vi "Flatten.vi"(8 "error in":errorcluster, 9 "Data":T1) -> (0 "error out":errorcluster, 2 "Buffer":u8[](array[numeric]) format="%.0x")   [LabVIEW 2020, in "TcpPayload.lvlib"]
uses:
  TcpPayload.lvlib
  Data.ctl
  lv-protoc/LV-Proto/LV-Proto.lvlib
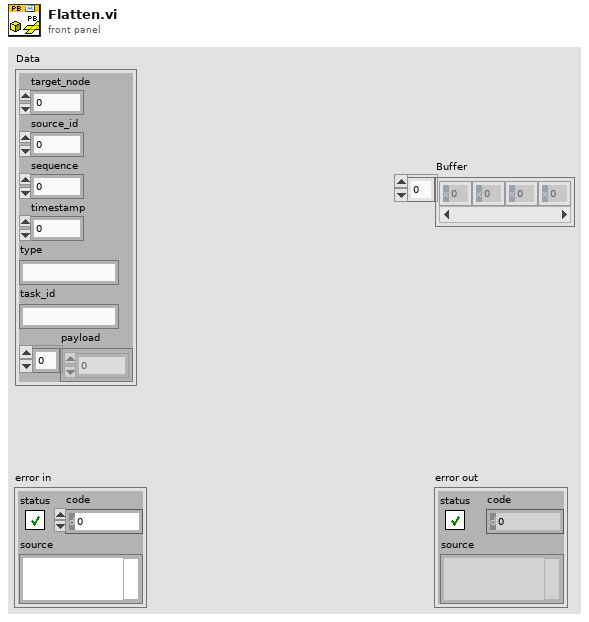
[diagram p1: front panel]
types:
  T1 = typedef "TcpPayload.lvlib/Data.ctl" = cluster{"target_node":u32, "source_id":u32, "sequence":u32, "timestamp":u64, "type":string, "task_id":string, "payload":u8[]}
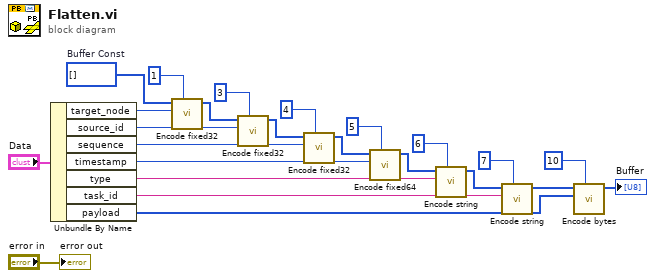
[diagram p0: block diagram]
diagram:
  w22 = u8[] []  # Buffer Const
  n1 = Unbundle By Name("Data") -> ("target_node"=w20:u32, "source_id"=w17:u32, "sequence"=w14:u32, "timestamp"=w11:u64, "type"=w8:string, "task_id"=w5:string, "payload"=w2:u8[])
  n2 = call "Encode fixed32.vi"("Field Number"=1, "fixed32"=w20, "Buffer in"=w22) -> ("Buffer"=w19:u8[])  [unwired: 8 in]
  n3 = call "Encode fixed32.vi"("Field Number"=3, "fixed32"=w17, "Buffer in"=w19) -> ("Buffer"=w16:u8[])  [unwired: 8 in]
  n4 = call "Encode fixed32.vi"("Field Number"=4, "fixed32"=w14, "Buffer in"=w16) -> ("Buffer"=w13:u8[])  [unwired: 8 in]
  n5 = call "Encode fixed64.vi"("Field Number"=5, "fixed64"=w11, "Buffer in"=w13) -> ("Buffer"=w10:u8[])  [unwired: 8 in]
  n6 = call "Encode string.vi"("Field Number"=6, "string"=w8, "Buffer in"=w10) -> ("Buffer"=w7:u8[])  [unwired: 8 in]
  n7 = call "Encode string.vi"("Field Number"=7, "string"=w5, "Buffer in"=w7) -> ("Buffer"=w4:u8[])  [unwired: 8 in]
  n8 = call "Encode bytes.vi"("Field Number"=10, "bytes"=w2, "Buffer in"=w4) -> ("Buffer"=→"Buffer":u8[])  [unwired: 8 in]
  "error out" <- "error in"
